vi "Create.vi"(8 "error in (no error)":errorcluster, 10 "Waveform Settings":T1, 11 "Waveform Factory in":refnum<class "Waveform Factory.lvclass">) -> (0 "error out":errorcluster, 2 "Waveform":refnum<class "Waveform.lvclass">, 3 "Waveform Factory out":refnum<class "Waveform Factory.lvclass">)   [LabVIEW 2016, in "Waveform Factory.lvclass"]
uses:
  Waveform Factory.lvclass
  Waveform/Waveform.lvclass
  Typedefs/WaveformSettings.ctl
  Typedefs/WaveformTypes.ctl
  Waveform Generator/Waveform Generator.lvclass
  C:/CODE/ts_HPMT/Model/Waveforms/Waveform/Waveform.lvclass
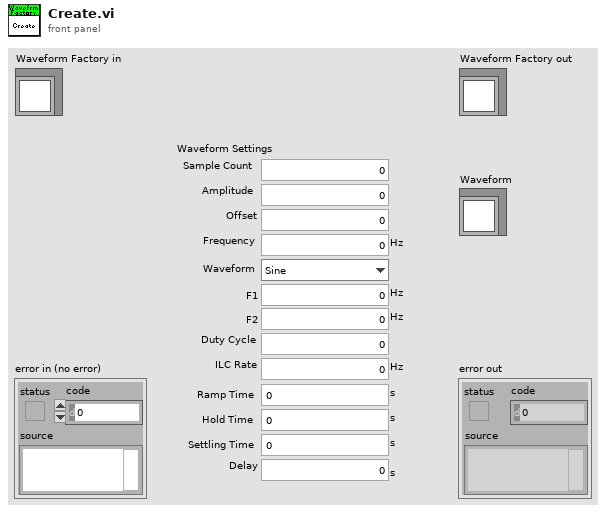
[diagram p1: front panel]
types:
  T1 = typedef "WaveformSettings.ctl" = cluster{"Sample Count":u32, "Amplitude":dbl, "Offset":dbl, "Frequency":dbl[unit], "Waveform":T2, "F1":dbl[unit], "F2":dbl[unit], "Duty Cycle":dbl, "ILC Rate":dbl[unit], "Ramp Time":dbl[unit], "Hold Time":dbl[unit], "Settling Time":dbl[unit], "Delay":dbl[unit]}
  T2 = typedef "WaveformTypes.ctl" = enum16{"Sine", "Triangle", "Square", "Sawtooth", "Chirp", "Gaussian", "Trapezoid", "Constant"}
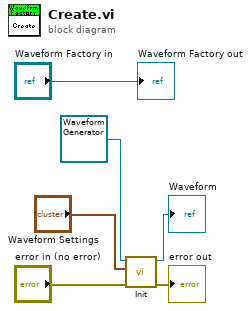
[diagram p0: block diagram]
diagram:
  n1 = call "Init.vi"("error in (no error)"="error in (no error)", "Waveform Settings"="Waveform Settings", "Waveform Generator in"=refnum<class "Waveform Generator.lvclass"> refnum ("Waveform Generator.lvclass")) -> ("error out"=→"error out":errorcluster, "Waveform Generator out"=→"Waveform":refnum<class "Waveform Generator.lvclass">)  [unwired: 7 in]
  "Waveform Factory out" <- "Waveform Factory in"
